vi "getBooleanValue.vi"(7 "Name":string, 8 "error in (no error)":errorcluster, 11 "tBSONDocument in":refnum<class "tBSONDocument.lvclass">) -> (0 "error out":errorcluster, 2 "Value":bool, 3 "tBSONDocument out":refnum<class "tBSONDocument.lvclass">)   [LabVIEW 2013, in "BSON.lvlib" / "tBSONDocument.lvclass"]
doc: "Retrieves a boolean from a BSON document."
uses:
  tBSONDocument.lvclass
  BSONElements/tBSONBoolean/tBSONBoolean.lvclass
  BSONElements/tBSONBoolean/getValue.vi
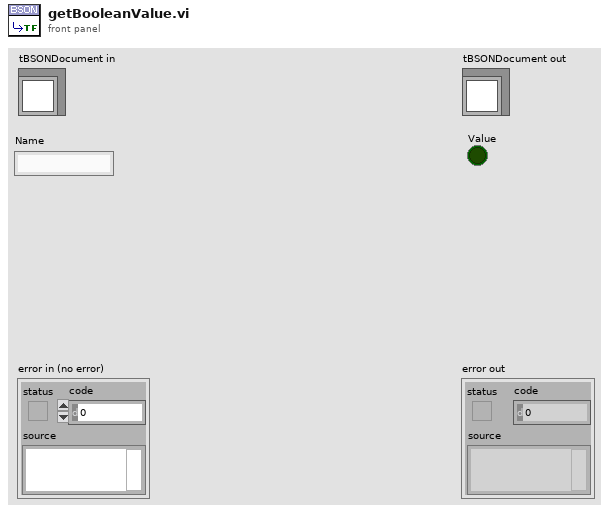
[diagram p1: front panel]
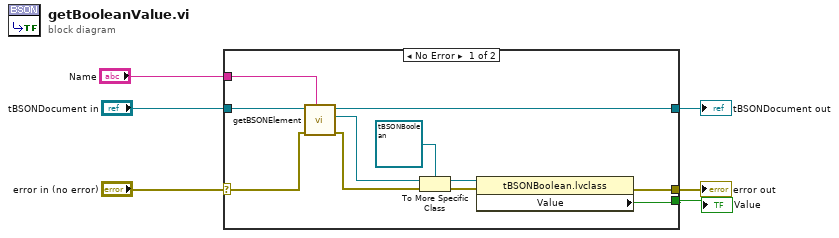
[diagram p0: block diagram]
diagram:
  n1 = case shown="No Error" "error in (no error)" {
    selector: "error in (no error)" -> [w11 w19]
    tunnel: [w10 w19] -> w5
    tunnel: [w12 w18] -> w3
    tunnel: "tBSONDocument in" -> [w13 w18]
    tunnel: "Name" -> [w7 _]
    tunnel: [w8 _] -> w1
    frame No Error {
      n2 = call "getBSONElement.vi"("Name"=w7, "error in (no error)"=w11, "tBSONDocument in"=w13) -> ("error out"=w15:errorcluster, "Element"=w14:refnum<class "tBSONElement.lvclass">, "tBSONDocument out"=w12:refnum<class "tBSONDocument.lvclass">)  [unwired: 6 in]
      n3 = To More Specific Class(target class=refnum<class "tBSONBoolean.lvclass"> refnum ("BSON.lvlib:tBSONBoolean.lvclass"), reference=w14, error in=w15) -> (specific class reference=w16:refnum<class "tBSONBoolean.lvclass">, error out=w17:errorcluster)
      n4 = property class="tBSONBoolean.lvclass"(reference=w16, error in=w17) -> (error out=w10:errorcluster, "Value"=w8:bool)  [unwired: 1 out]
    }
    frame Error {
    }
  }
  "error out" <- w5
  "tBSONDocument out" <- w3
  "Value" <- w1
